vi "Get Model(s) Config File.vi"(8 "Error In":errorcluster, 11 "eHS Matrix Generation Session Ref In":refnum<data-value>) -> (0 "Error Out":errorcluster, 2 "Model(s) Config File Path":path, 3 "eHS Matrix Generation Session Ref Out":refnum<data-value>)   [LabVIEW 2017]
uses:
  <vilib>/OPAL-RT/eHS Toolkit/eHS Matrix Generation/_Controls/eHS Matrix Generation Session.ctl
  <vilib>/OPAL-RT/eHS Toolkit/eHS Matrix Generation/_Controls/eHS Target Information.ctl
  <vilib>/OPAL-RT/eHS Toolkit/eHS Matrix Generation/_Controls/eHS Matrix Generation Parameters.ctl
  <vilib>/OPAL-RT/eHS Toolkit/eHS Matrix Generation/_Controls/eHS Circuit Analysis Data.ctl
  <vilib>/OPAL-RT/eHS Toolkit/eHS Matrix Generation/_Controls/eHS Core Settings.ctl
  <vilib>/OPAL-RT/eHS Toolkit/eHS Matrix Generation/_Controls/eHS Form Factor.ctl
  <vilib>/OPAL-RT/eHS Toolkit/eHS Matrix Generation/_Controls/eHS Core Index.ctl
  <vilib>/OPAL-RT/eHS Toolkit/eHS Matrix Generation/_Controls/eHS Model Information.ctl
  <vilib>/OPAL-RT/eHS Toolkit/eHS Matrix Generation/eHS Matrix Generation.lvlib
panel:
  in  "OK Button":bool
  in  "Model(s) Config File Path (INI File Only)":path
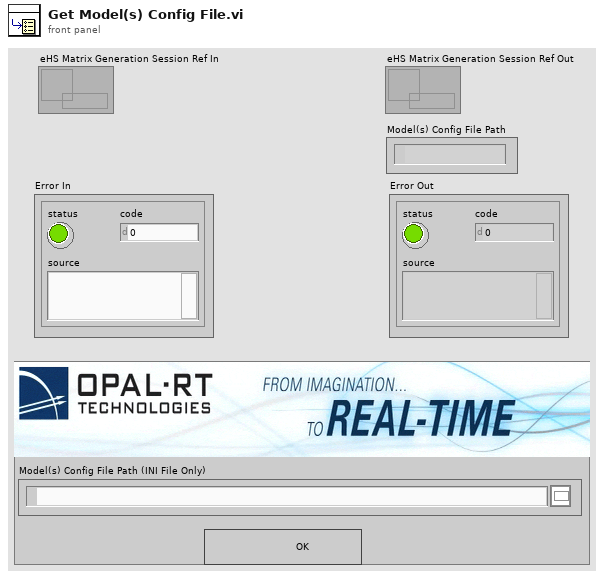
[diagram p1: front panel]
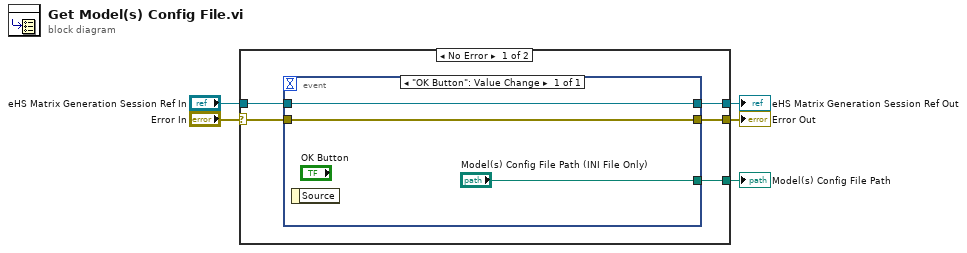
[diagram p0: block diagram]
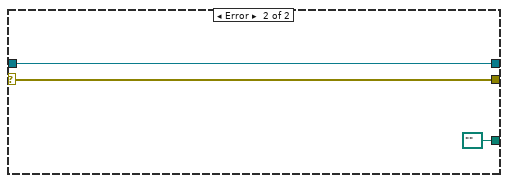
[diagram p2: hidden frame]
diagram:
  n1 = case shown="No Error" "Error In" {
    selector: "Error In" -> [w6 w16]
    tunnel: [w7 w16] -> w4
    tunnel: [w9 w15] -> w2
    tunnel: "eHS Matrix Generation Session Ref In" -> [w8 w15]
    tunnel: [w10 path "" ("Model(s) Config File Path (INI File Only)")] -> w3
    frame No Error {
      n2 = event shown="[0] \"OK Button\": Value Change" {
        selector: _ -> [_]
        dyn-events: _ -> [_]
        timeout: _ -> [_]
        tunnel: ["Model(s) Config File Path (INI File Only)"] -> w10
        tunnel: [w12] -> w9
        tunnel: w8 -> [w12]
        tunnel: [w11] -> w7
        tunnel: w6 -> [w11]
        event "OK Button": Value Change {
          n3 = event-data() -> ()  [unwired: 1 in, 1 out]
        }
      }
    }
    frame Error {
    }
  }
  "Error Out" <- w4
  "Model(s) Config File Path" <- w3
  "eHS Matrix Generation Session Ref Out" <- w2
